vi "Read Measurement.vi"(6 "error in":errorcluster, 9 "VISA resource name":refnum<visa-resource-name>) -> (0 "error out":errorcluster, 2 "Measurement":dbl, 3 "VISA resource name out":refnum<visa-resource-name>)   [LabVIEW 2023, in "Aim TTi 1908P DMM.lvlib"]
uses:
  Aim TTi 1908P DMM.lvlib
  19e38209-455c-425b-9d7c-0b824d84d338.vi
panel:
  out "read buffer":string
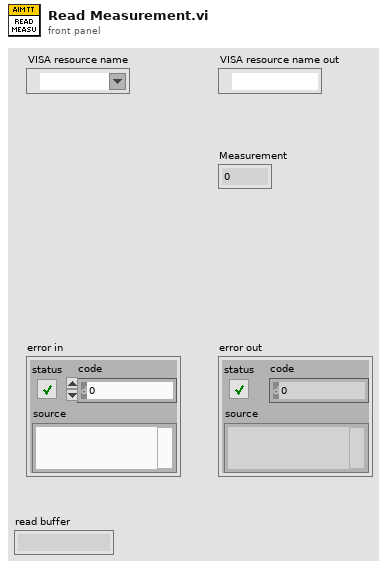
[diagram p1: front panel]
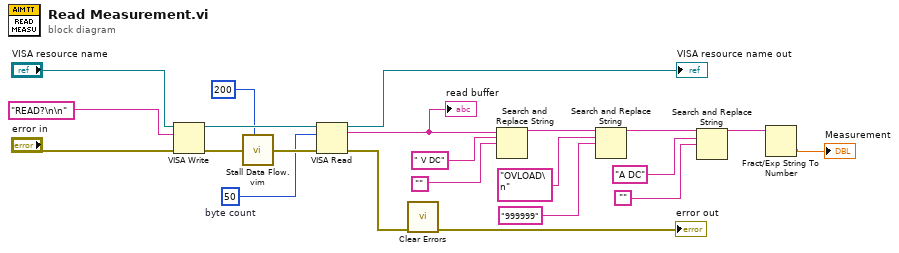
[diagram p0: block diagram]
diagram:
  w14 = u32 50  # byte count
  n1 = VISA Write(VISA resource name="VISA resource name", write buffer="READ?\n\n", error in (no error)="error in") -> (VISA resource name out=w22:refnum<visa-resource-name>, error out=w21:errorcluster)  [unwired: 1 out]
  n2 = call "Stall Data Flow.vim"("value in"=w21, "milliseconds to wait"=u32 200) -> ("value out"=w20:errorcluster)  [unwired: 1 out]
  n3 = VISA Read(VISA resource name=w22, byte count=w14, error in (no error)=w20) -> (VISA resource name out=→"VISA resource name out":refnum<visa-resource-name>, read buffer=w2:string, error out=w15:errorcluster)  [unwired: 1 out]
  "read buffer" <- w2
  n4 = call <vilib>:"Clear Errors.vi"("error in (no error)"=w15) -> ("error out"=→"error out":errorcluster)  [unwired: 5 in, 1 out]
  n5 = Search and Replace String(input string=w2, search string=" V DC", replace string="") -> (result string=w10:string)  [unwired: 5 in, 3 out]
  n6 = Search and Replace String(input string=w10, search string="OVLOAD\n", replace string="999999" ("replace string (\"\")")) -> (result string=w6:string)  [unwired: 5 in, 3 out]
  n7 = Search and Replace String(input string=w6, search string="A DC", replace string="") -> (result string=w5:string)  [unwired: 5 in, 3 out]
  n8 = Fract/Exp String To Number(string=w5) -> (number=→"Measurement":dbl)  [unwired: 3 in, 1 out]
